vi "Timer Off Delay.vi"(8 "error in":errorcluster, 10 "preset time (ms)":i32=1000, 11 "input":bool) -> (0 "error out":errorcluster, 2 "elapsed time (ms)":i32, 3 "output":bool)   [LabVIEW 2017, in "NI_FunctionBlock Libraries.lvlib"]
uses:
  <vilib>/functionblocks/NI_FunctionBlock Libraries.lvlib
  <vilib>/ptbypt/NI_PtbyPt.lvlib
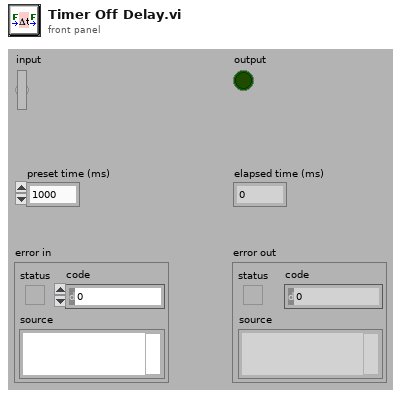
[diagram p1: front panel]
types:
  T1 = enum16{"Initialize", "Waiting for rising edge", "Waiting for falling edge", "Counting down"}
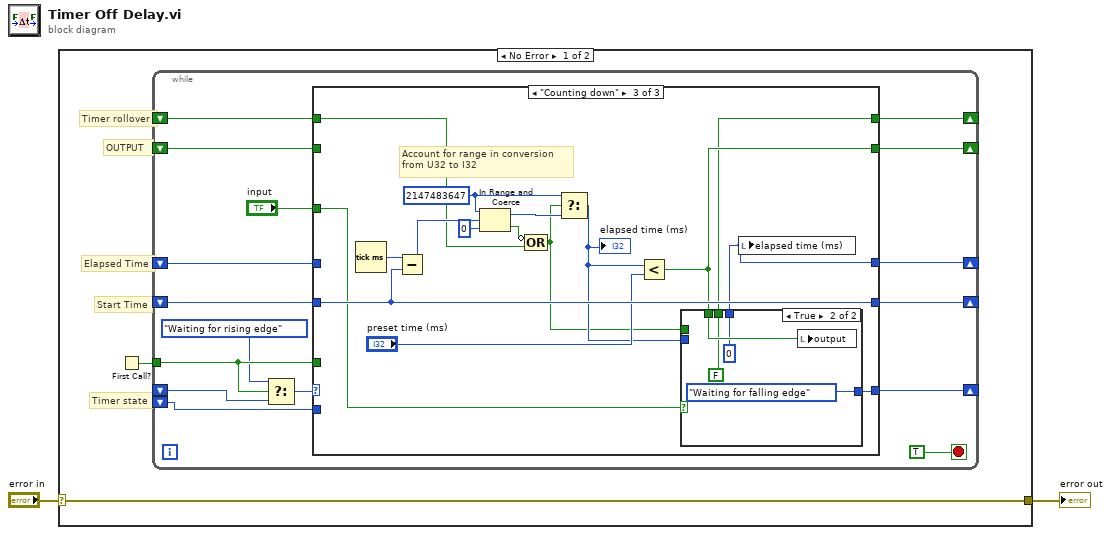
[diagram p0: block diagram]
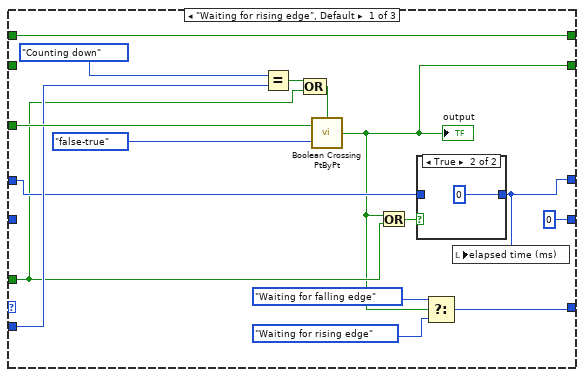
[diagram p2: hidden frame]
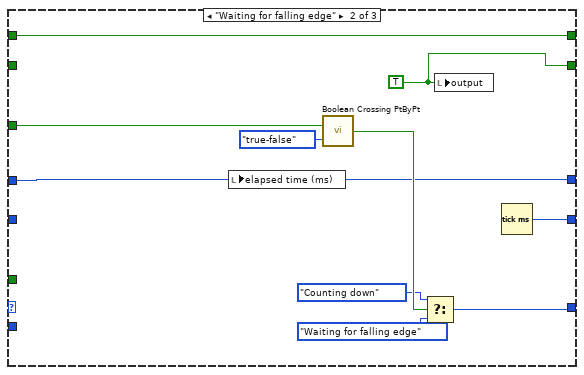
[diagram p4: hidden frame]
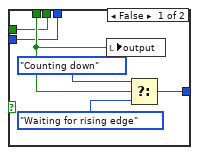
[diagram p5: hidden frame]
diagram:
  n1 = case shown="No Error" "error in" {
    selector: "error in" -> [w3 w75]
    tunnel: [w3 w75] -> w1
    frame No Error {
      # "Timer rollover"
      # "Timer state"
      # "Start Time"
      # "Elapsed Time"
      # "OUTPUT"
      n2 = First Call?() -> (First Call?: T/F=w4:bool)
      n3 = while {
        shift-right: [w19] -> _
        shift-left: _ -> [w14]
        shift-right: [w18] -> _
        shift-left: _ -> [w17]
        tunnel: w4 -> [w12]
        shift-left: _ -> [w13]
        shift-right: [w11] -> _
        shift-left: _ -> [w10]
        shift-right: [w9] -> _
        shift-left: _ -> [w8]
        shift-right: [w6] -> _
        shift-left: _ -> [w5]
        stop <- TRUE stop-if-true
        n4 = Select(t=T1."Waiting for rising edge", s=w12, f=w14) -> (s? t:f=w15:T1)
        n5 = case shown="\"Counting down\"" w15 {
          tunnel: "input" -> [w36 w48 w60]
          tunnel: [w35 w45 w61] -> w19
          tunnel: [u32 0 ("millisecond timer value") w42 w63] -> w18
          tunnel: w17 -> [_ _ w63]
          tunnel: w13 -> [w30 _ _]
          tunnel: w12 -> [w24 _ _]
          tunnel: [w23 w41 w59] -> w11
          tunnel: w10 -> [_ _ _]
          tunnel: [w26 w40 w58] -> w9
          tunnel: w8 -> [w25 w40 _]
          tunnel: [w21 w39 w50] -> w6
          tunnel: w5 -> [w21 w39 w51]
          frame "Waiting for rising edge", Default {
            n6 = Equal?(x=T1."Counting down", y=w30) -> (x = y?=w28:bool)
            n7 = Compound Arithmetic op=OR(w28, w24) -> (w27:bool)
            n8 = call <vilib>:"Boolean Crossing PtByPt.vi"("initialize"=w27, "direction"=enum16{"either", "false-true", "true-false"}."false-true", "input"=w36) -> ("crossing"=w23:bool)
            "output" <- w23
            n9 = Or(x=w23, y=w24) -> (x .or. y?=w22:bool)
            n10 = case shown="True" w22 {
              tunnel: [w37 0 ("ET (ms)")] -> w26
              tunnel: w25 -> [w37 _]
              frame False {
              }
              frame True {
              }
            }
            n11 = Select(t=T1."Waiting for falling edge", s=w23, f=T1."Waiting for rising edge") -> (s? t:f=w35:T1)
            n12 = local write "elapsed time (ms)"(w26) -> ()
          }
          frame "Waiting for falling edge" {
            w41 = TRUE ("Q")
            n13 = local write "elapsed time (ms)"(w40) -> ()
            n14 = call <vilib>:"Boolean Crossing PtByPt.vi"("direction"=enum16{"either", "false-true", "true-false"}."true-false", "input"=w48) -> ("crossing"=w46:bool)  [unwired: 1 in]
            n15 = Select(t=T1."Counting down", s=w46, f=T1."Waiting for falling edge") -> (s? t:f=w45:T1)
            n16 = local write "output"(w41) -> ()
            n17 = Tick Count (ms)() -> (millisecond timer value=w42:u32)
          }
          frame "Counting down" {
            w55 = u32 2147483647 ("upper limit")
            # "Account for range in conversion\nfrom U32 to I32"
            n18 = Tick Count (ms)() -> (millisecond timer value=w64:u32)
            n19 = Subtract(x=w64, y=w63) -> (x-y=w53:u32)
            n20 = In Range and Coerce(upper limit=w55, x=w53, lower limit=u32 0) -> (coerced(x)=w54:u32, In Range?=w56:bool)
            n21 = Compound Arithmetic op=OR(invert w56, w51) -> (w49:bool)
            n22 = Select(t=w55, s=w49, f=w54) -> (s? t:f=w52:u32)
            "elapsed time (ms)" <- w52
            n23 = Less?(x=w52, y="preset time (ms)") -> (x < y?=w59:bool)
            n24 = case shown="True" w60 {
              tunnel: [w70 T1."Waiting for falling edge"] -> w61
              tunnel: w59 -> [w69 w74]
              tunnel: w52 -> [w66 _]
              tunnel: [w66 u32 0] -> w58
              tunnel: [w65 FALSE] -> w50
              tunnel: w49 -> [w65 _]
              frame False {
                n25 = local write "output"(w69) -> ()
                n26 = Select(t=T1."Counting down", s=w69, f=T1."Waiting for rising edge") -> (s? t:f=w70:T1)
              }
              frame True {
                n27 = local write "output"(w74) -> ()
              }
            }
            n28 = local write "elapsed time (ms)"(w58) -> ()
          }
        }
      }
    }
    frame Error {
    }
  }
  "error out" <- w1
